vi "setRootIcons.vi"(8 "error in (no error)":errorcluster, 11 "reference":refnum<vi>) -> (0 "error out":errorcluster, 3 "reference out":refnum<vi>)   [LabVIEW 2010]
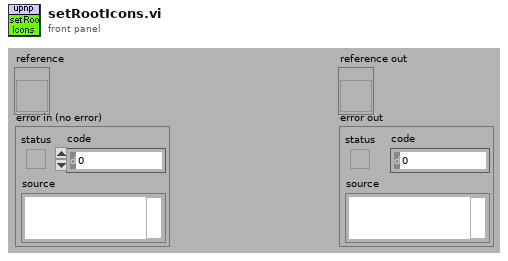
[diagram p1: front panel]
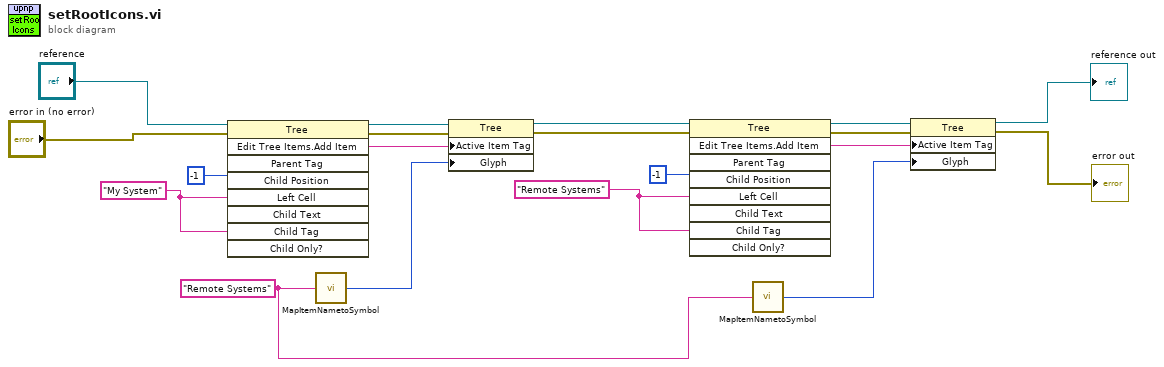
[diagram p0: block diagram]
diagram:
  w3 = "Remote Systems" ("Item Name")
  w4 = "Remote Systems" ("Left Cell String")
  w6 = "My System" ("Left Cell String")
  n1 = invoke class="Tree" method="Edit Tree Items.Add Item"(reference="reference", error in="error in (no error)", "Child Position"=-1, "Left Cell"=w6, "Child Tag"=w6) -> (reference out=w18:refnum<vi>, error out=w17:errorcluster, "Edit Tree Items:Add Item"=w16:string)  [unwired: 4 in, 6 out]
  n2 = call "MapItemNametoSymbol.vi"("Item Name"=w3) -> ("Symbol Index"=w15:i32)  [unwired: 4 out]
  n3 = property class="Tree"(reference=w18, error in=w17, "Active Item Tag"=w16, "Glyph"=w15) -> (reference out=w8:refnum<vi>, error out=w7:errorcluster)
  n4 = invoke class="Tree" method="Edit Tree Items.Add Item"(reference=w8, error in=w7, "Child Position"=-1, "Left Cell"=w4, "Child Tag"=w4) -> (reference out=w11:refnum<vi>, error out=w10:errorcluster, "Edit Tree Items:Add Item"=w9:string)  [unwired: 4 in, 6 out]
  n5 = call "MapItemNametoSymbol.vi"("Item Name"=w3) -> ("Symbol Index"=w5:i32)  [unwired: 4 out]
  n6 = property class="Tree"(reference=w11, error in=w10, "Active Item Tag"=w9, "Glyph"=w5) -> (reference out=→"reference out":refnum<vi>, error out=→"error out":errorcluster)
